vi "Service Location FGV.vi"(8 "error in":errorcluster, 9 "location unique id in":u64, 10 "resolve service request":T2, 11 "action":T1) -> (0 "error out":errorcluster, 1 "location unique id out":u64, 3 "service location":T3)   [LabVIEW 2020, in "Measurement Plugin Discovery V1.lvlib"]
uses:
  Measurement Plugin Discovery V1.lvlib
  Resolve Service.vi
  Measurement Plugin Discovery Client/RPC Messages/ni_measurementlink_discovery_v1_ServiceLocation.ctl
  Measurement Plugin Discovery Client/Measurement Plugin Discovery Client.lvlib
  Measurement Plugin Discovery Client/RPC Messages/ni_measurementlink_discovery_v1_ResolveServiceRequest.ctl
  TypeDefs/Service Location FGV Action.ctl
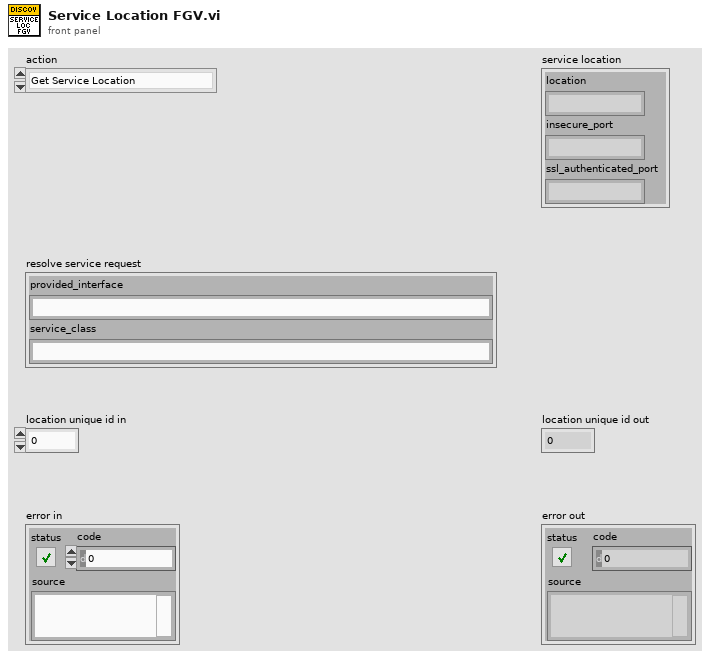
[diagram p1: front panel]
types:
  T1 = typedef "Measurement Plugin Discovery V1.lvlib/Service Location FGV Action.ctl" = enum16{"Get Service Location", "Reresolve Service Location"}
  T2 = typedef "Measurement Plugin Discovery Client.lvlib/ni_measurementlink_discovery_v1_ResolveServiceRequest.ctl" = cluster{"provided_interface":string, "service_class":string}
  T3 = typedef "Measurement Plugin Discovery Client.lvlib/ni_measurementlink_discovery_v1_ServiceLocation.ctl" = cluster{"location":string, "insecure_port":string, "ssl_authenticated_port":string}
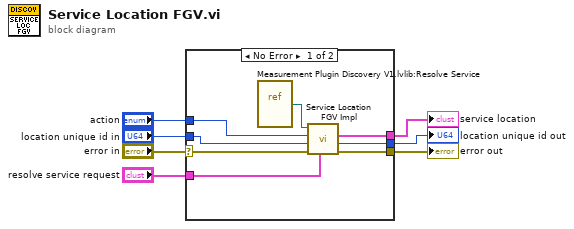
[diagram p0: block diagram]
diagram:
  n1 = case shown="No Error" "error in" {
    selector: "error in" -> [w11 w16]
    tunnel: [w10 w16] -> w5
    tunnel: [w9 _] -> w7
    tunnel: "resolve service request" -> [w12 _]
    tunnel: "action" -> [w14 _]
    tunnel: [w8 _] -> w2
    tunnel: "location unique id in" -> [w13 _]
    frame No Error {
      n2 = vi-ref "Measurement Plugin Discovery V1.lvlib:Resolve Service.vi"() -> (w15:refnum<vi>)
      n3 = call "Service Location FGV Impl.vi"("resolve service request"=w12, "error in"=w11, "location unique id in"=w13, "action"=w14, "resolve vi reference"=w15) -> ("error out"=w10:errorcluster, "location unique id out"=w8:u64, "service location"=w9:T3)  [unwired: 4 in]
    }
    frame Error {
    }
  }
  "service location" <- w7
  "error out" <- w5
  "location unique id out" <- w2
